vi "hardware_close_hardware.vi"(8 "error in (no error)":errorcluster, 11 "hydraharp in":refnum<class "hydraharp.lvclass">) -> (0 "error out":errorcluster, 3 "hydraharp out":refnum<class "hydraharp.lvclass">)   [LabVIEW 2015, in "hydraharp.lvclass"]
uses:
  hydraharp.lvclass
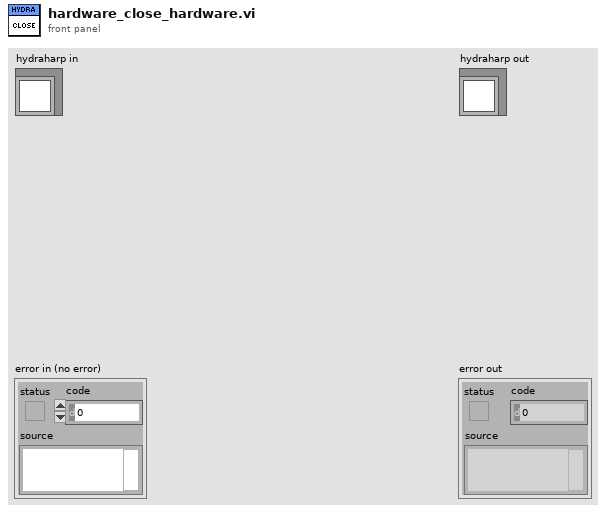
[diagram p1: front panel]
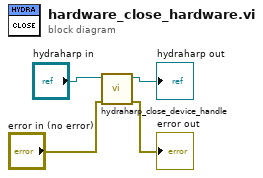
[diagram p0: block diagram]
diagram:
  n1 = call "hydraharp_close_device_handle.vi"("error in (no error)"="error in (no error)", "hydraharp in"="hydraharp in") -> ("error out"=→"error out":errorcluster, "hydraharp out"=→"hydraharp out":refnum<class "hydraharp.lvclass">)  [unwired: 8 in]
